vi "Initialize.vi"(8 "error in (no error)":errorcluster, 11 "Mettler Settings in":T1) -> (0 "error out":errorcluster, 2 "No Scale Connected":bool, 3 "Mettler Settings out":T1)   [LabVIEW 2018, in "Mettler Toledo.lvlib"]
uses:
  Mettler Toledo.lvlib
  Controls/Settings Cluster.ctl
  <vilib>/Instr/_visa.llb/VISA Configure Serial Port (Instr).vi
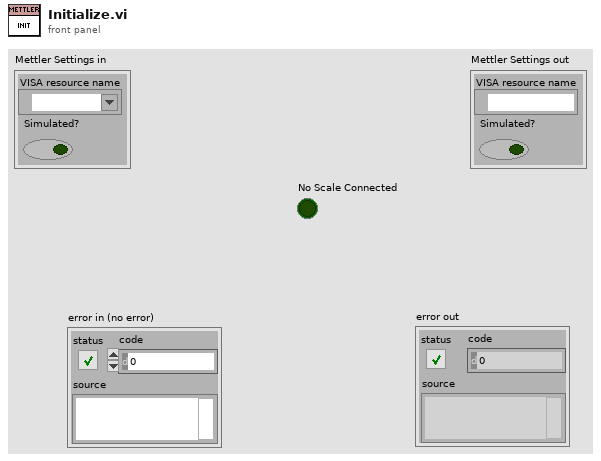
[diagram p1: front panel]
types:
  T1 = typedef "Mettler Toledo.lvlib/Settings Cluster.ctl" = cluster{"VISA resource name":refnum<visa-resource-name>, "Simulated?":bool}
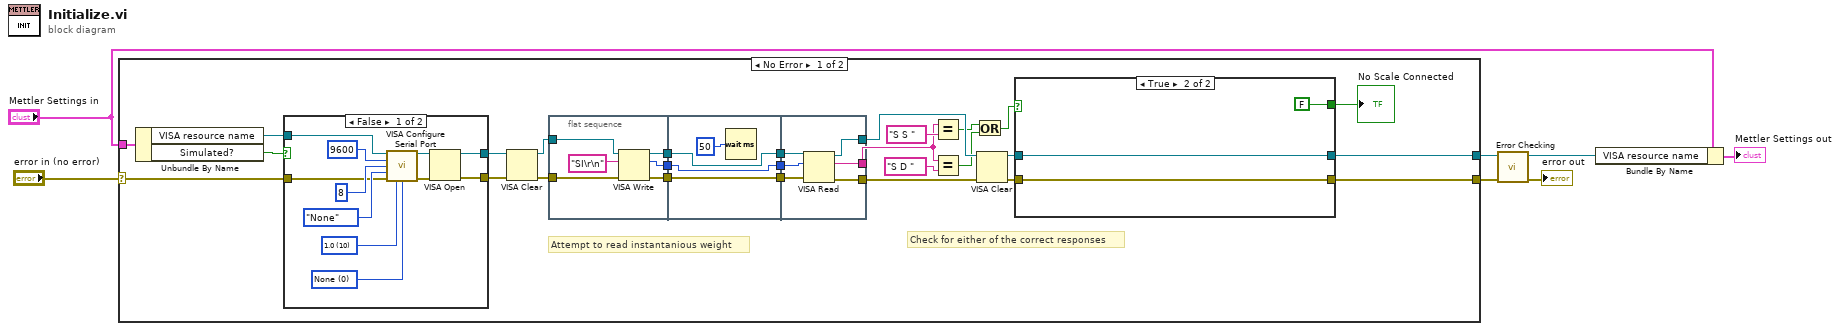
[diagram p0: block diagram]
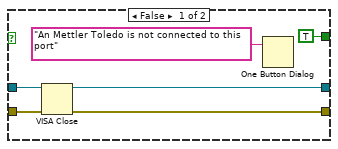
[diagram p2: hidden frame]
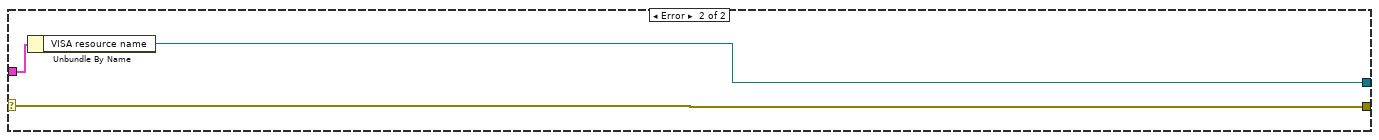
[diagram p4: hidden frame]
diagram:
  n1 = case shown="No Error" "error in (no error)" {
    selector: "error in (no error)" -> [w34 w74]
    tunnel: "Mettler Settings in" -> [w32 w73]
    tunnel: [w28 w74] -> w2
    tunnel: [w29 w72] -> w4
    frame No Error {
      # "Check for either of the correct responses"
      # "Attempt to read instantanious weight"
      n2 = Unbundle By Name(w32) -> ("VISA resource name"=w31:refnum<visa-resource-name>, "Simulated?"=w33:bool)
      n3 = case shown="False" w33 {
        tunnel: w34 -> [w63 w71]
        tunnel: [w59 w71] -> w20
        tunnel: [w60 w70] -> w21
        tunnel: w31 -> [w61 w70]
        frame False {
          w65 = u16 0 items=["None", "XON/XOFF", "RTS/CTS", "XON/XOFF & RTS/CTS", "DTR/DSR", "XON/XOFF & DTR/DSR"] ("flow control (0:none)")
          w66 = u16 10 items=["1.0"=10, "1.5"=15, "2.0"=20] ("stop bits (10: 1 bit)")
          n4 = call-poly "VISA Configure Serial Port"("VISA resource name"=w61, "baud rate (9600)"=u32 9600, "data bits (8)"=u16 8, "parity (0:none)"=enum16{"None", "Odd", "Even", "Mark", "Space"}."None", "error in (no error)"=w63, "stop bits (10: 1 bit)"=w66, "flow control (0:none)"=w65) -> ("VISA resource name out"=w62:refnum<visa-resource-name>, "error out"=w64:errorcluster)  [unwired: 7 in]
          n5 = VISA Open(error in (no error)=w64, VISA resource name=w62) -> (VISA resource name=w60:refnum<visa-resource-name>, error out=w59:errorcluster)  [unwired: 3 in]
        }
        frame True {
        }
      }
      n6 = VISA Clear(VISA resource name=w21, error in (no error)=w20) -> (VISA resource name out=w19:refnum<visa-resource-name>, error out=w18:errorcluster)
      n7 = flat-sequence {
        tunnel: w18 -> [w40]
        tunnel: w19 -> [w39]
        tunnel: [w37] -> w27
        tunnel: [w36] -> w25
        tunnel: [w35] -> w16
        tunnel: w27 -> [w44]
        tunnel: [w44] -> w26
        tunnel: w25 -> [w43]
        tunnel: [w43] -> w24
        tunnel: [w41] -> w17
        tunnel: w16 -> [w41]
        tunnel: [w50] -> w14
        tunnel: [w49] -> w12
        tunnel: [w48] -> w15
        tunnel: w26 -> [w47]
        tunnel: w24 -> [w46]
        tunnel: w17 -> [w45]
        frame #0 {
          n8 = VISA Write(VISA resource name=w39, write buffer="SI\r\n", error in (no error)=w40) -> (VISA resource name out=w37:refnum<visa-resource-name>, return count=w35:u32, error out=w36:errorcluster)
        }
        frame #1 {
          n9 = Wait (ms)(milliseconds to wait=u32 50) -> ()  [unwired: 1 out]
        }
        frame #2 {
          n10 = VISA Read(VISA resource name=w47, byte count=w45, error in (no error)=w46) -> (VISA resource name out=w48:refnum<visa-resource-name>, read buffer=w49:string, error out=w50:errorcluster)  [unwired: 1 out]
        }
      }
      n11 = Equal?(x=w12, y="S S ") -> (x = y?=w11:bool)
      n12 = Equal?(x=w12, y="S D ") -> (x = y?=w10:bool)
      n13 = Or(x=w11, y=w10) -> (x .or. y?=w9:bool)
      n14 = VISA Clear(VISA resource name=w15, error in (no error)=w14) -> (VISA resource name out=w23:refnum<visa-resource-name>, error out=w22:errorcluster)
      n15 = case shown="True" w9 {
        tunnel: w23 -> [w53 w58]
        tunnel: w22 -> [w54 w57]
        tunnel: [w53 w58] -> w29
        tunnel: [w52 w57] -> w28
        tunnel: [TRUE FALSE] -> w8
        frame False {
          n16 = VISA Close(VISA resource name=w53, error in (no error)=w54) -> (error out=w52:errorcluster)
          n17 = One Button Dialog(message="An Mettler Toledo is not connected to this port") -> ()  [unwired: 1 in, 1 out]
        }
        frame True {
        }
      }
      "No Scale Connected" <- w8
    }
    frame Error {
      n18 = Unbundle By Name(w73) -> ("VISA resource name"=w72:refnum<visa-resource-name>)
    }
  }
  n19 = call "Error Checking.vi"("error in (no error)"=w2, "VISA resource name"=w4) -> ("error out"=→"error out":errorcluster, "VISA resource name"=w3:refnum<visa-resource-name>)  [unwired: 7 in, 1 out]
  n20 = Bundle By Name(cluster="Mettler Settings in", "VISA resource name"=w3) -> (→"Mettler Settings out":T1)
